vi "MGI Get Tree Tag Children.vi"(9 "Tag (\"\": root items)":string, 10 "error in (no error)":errorcluster, 11 "Tree Ref":refnum<vi>) -> (1 "Child Tag[]":string[](array[string]), 2 "error out":errorcluster, 3 "Tree Ref (Dup)":refnum<vi>)   [LabVIEW 2020]
doc: "Get all child tags of the specified tag for the specified tree control.\n\nAuthored by Shawn D. Walpole\nsupport@mooregoodideas.com\nwww.mooregoodideas.com\n\nCopyright (c) 2010, Moore Good Ideas, Inc.\n\nAll rights reserved.\n\nRedistribution and use in source and binary forms, with or without modification, are permitted provided that the following conditions are met:\n\n * Redistributions of source code must retain the above copyright notice, this list of conditions and the following disclaimer.\n * Redistributions in binary form must reproduce the above copyright notice, this list of conditions and the following disclaimer in the documentation and/or other materials provided with the distribution.\n * Neither the name of Moore Good Ideas, Inc. nor the names of its contributors may be used to endorse or promote products derived from this software without specific prior written permission.\n\nTHIS SOFTWARE IS PROVIDED BY THE COPYRIGHT HOLDERS AND CONTRIBUTORS \"AS IS\" AND ANY EXPRESS OR IMPLIED WARRANTIES, INCLUDING, BUT NOT LIMITED TO, THE IMPLIED WARRANTIES OF MERCHANTABILITY AND FITNESS FOR A PARTICULAR PURPOSE ARE DISCLAIMED. IN NO EVENT SHALL THE COPYRIGHT OWNER OR CONTRIBUTORS BE LIABLE FOR ANY DIRECT, INDIRECT, INCIDENTAL, SPECIAL, EXEMPLARY, OR CONSEQUENTIAL DAMAGES (INCLUDING, BUT NOT LIMITED TO, PROCUREMENT OF SUBSTITUTE GOODS OR SERVICES; LOSS OF USE, DATA, OR PROFITS; OR BUSINESS INTERRUPTION) HOWEVER CAUSED AND ON ANY THEORY OF LIABILITY, WHETHER IN CONTRACT, STRICT LIABILITY, OR TORT (INCLUDING NEGLIGENCE OR OTHERWISE) ARISING IN ANY WAY OUT OF THE USE OF THIS SOFTWARE, EVEN IF ADVISED OF THE POSSIBILITY OF SUCH DAMAGE."
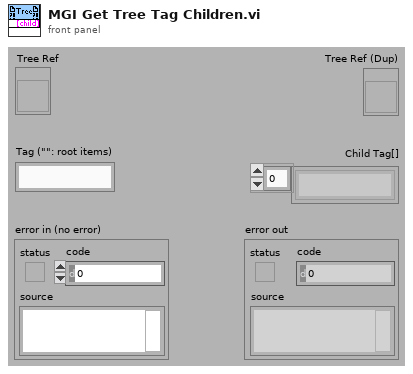
[diagram p1: front panel]
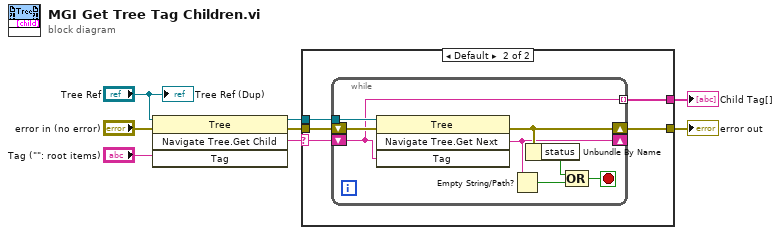
[diagram p0: block diagram]
diagram:
  n1 = invoke class="Tree" method="Navigate Tree.Get Child"(reference="Tree Ref", error in="error in (no error)", "Tag"="Tag (\"\": root items)") -> (reference out=w3:refnum<vi>, error out=w5:errorcluster, "Navigate Tree:Get Child"=w6:string)  [unwired: 1 in, 1 out]
  n2 = case shown="Default" w6 {
    selector: w6 -> [_ w14]
    tunnel: w5 -> [w9 w12]
    tunnel: [w9 w10] -> w4
    tunnel: w3 -> [_ w13]
    tunnel: [_ w11] -> w2
    frame "" {
    }
    frame Default {
      n3 = while {
        shift-right: [w16] -> _
        shift-left: w14 -> [w15]
        tunnel: w13 -> [w22]
        shift-right: [w17] -> w10
        shift-left: w12 -> [w21]
        tunnel: [w15] -> w11 mode=indexing
        stop <- w19 stop-if-true
        n4 = invoke class="Tree" method="Navigate Tree.Get Next"(reference=w22, error in=w21, "Tag"=w15) -> (error out=w17:errorcluster, "Navigate Tree:Get Next Item"=w16:string)  [unwired: 1 in, 2 out]
        n5 = Empty String/Path?(string/path=w16) -> (empty?=w20:bool)
        n6 = Unbundle By Name(w17) -> ("status"=w18:bool)
        n7 = Compound Arithmetic op=OR(w18, w20) -> (w19:bool)
      }
    }
  }
  "error out" <- w4
  "Child Tag[]" <- w2
  "Tree Ref (Dup)" <- "Tree Ref"
